vi "Measurement UI.vi"() -> ()   [LabVIEW 2021, in "crosstalk_Audio ADC.lvlib"]
uses:
  crosstalk_Audio ADC.lvlib
panel:
  out "MeasTable":string[][](table)
  in  "MeasGraphs":T1(tab)=enum."Time Domain"
  out "FreqDomainGraph":cluster{"f0":dbl, "df":dbl, "Spectrum":dbl[]}[](graph) caption="AC"
  out "TimeDomainGraph":waveform(dbl)[](graph) caption="AC"
  out "Time domain plot size":i32
  out "Spectrum plot size":i32
  out "dt":dbl
  out "t0":dbl
  out "df":dbl
  out "f0":dbl
  out "Time domain":dbl[](array[numeric])
  out "Spectrum":dbl[](array[numeric])
  out "Frequency 2":dbl
  out "Crosstalk":dbl
  out "Victim channel name":string
  out "Crosstalk waveform":dbl[](array[numeric])
  out "Frequency waveform":dbl[](array[numeric])
  in  "Victim channel resource name":string
  in  "Digital capture resource name":string
  in  "Configuration tab":enum32{"Protocol", "Measurement"}(tab)=enum."Measurement"
  in  "Frame sync edge for Channel 0":enum16{"Rising", "Falling"}(ring)=enum."Falling"
  in  "Channel count per frame":u8=2
  in  "Channel length":u16=32
  in  "Bit depth":u8=24
  in  "Channel 0 offset":u16=1
  in  "Endianness":enum16{"MSB First", "LSB First"}(ring)
  in  "Data Justification":enum16{"Left Justified", "Right Justified"}(ring) caption="Data justification"
  in  "Frame length":u16=64
  in  "Frame sync pulse width":u16=32
  in  "Bit clock edge sync":enum8{"Rising", "Falling"}(ring)=enum."Falling"
  in  "I2S":bool
  in  "LJ":bool
  in  "RJ":bool
  in  "TDM":bool
  in  "Analog source resource name":string(combo) caption="Resource Name"
  in  "Protocol capture resource name":string(combo) caption="Resource Name"
  in  "Channel Name":string
  in  "Full scale range":dbl=2.825 caption="FULL SCALE RANGE" format="%.3pV"
  in  "Weighting Filter":string(combo)="Linear"
  in  "Data line":u16 caption="Data Line"
  in  "Sample rate":dbl=44100.0 caption="Sample Rate" format="%#.6pHz"
  in  "Measurement settings":string="Measurement Settings"
  in  "Victim amplitude":dbl=1.0 caption="Amplitude" format="%#_6pdB"
  in  "Frequency":dbl=1000.0 format="%#_6pHz"
  in  "Victim channel":dbl=1.0 caption="Vicitim Channel" format="%#_6p"
  in  "Interferer channel":dbl caption="Interferer Channel" format="%#_6p"
  in  "Analog source":string="Analog source"
  in  "Digital capture":string="Digital capture"
  # "Protocols"
  # "PCM data configuration"
  # "Frame sync clock control"
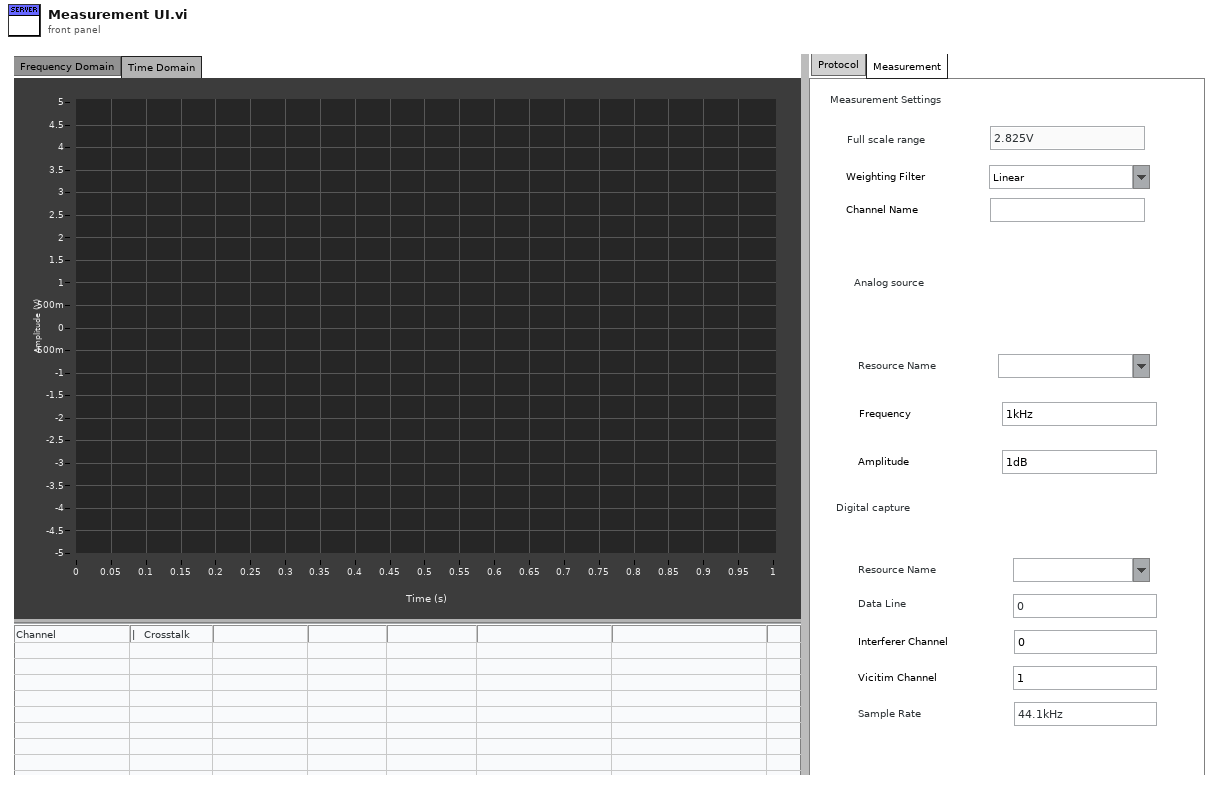
[diagram p1: front panel]
types:
  T1 = enum32{"Frequency Domain", "Time Domain", "Hidden Controls"}
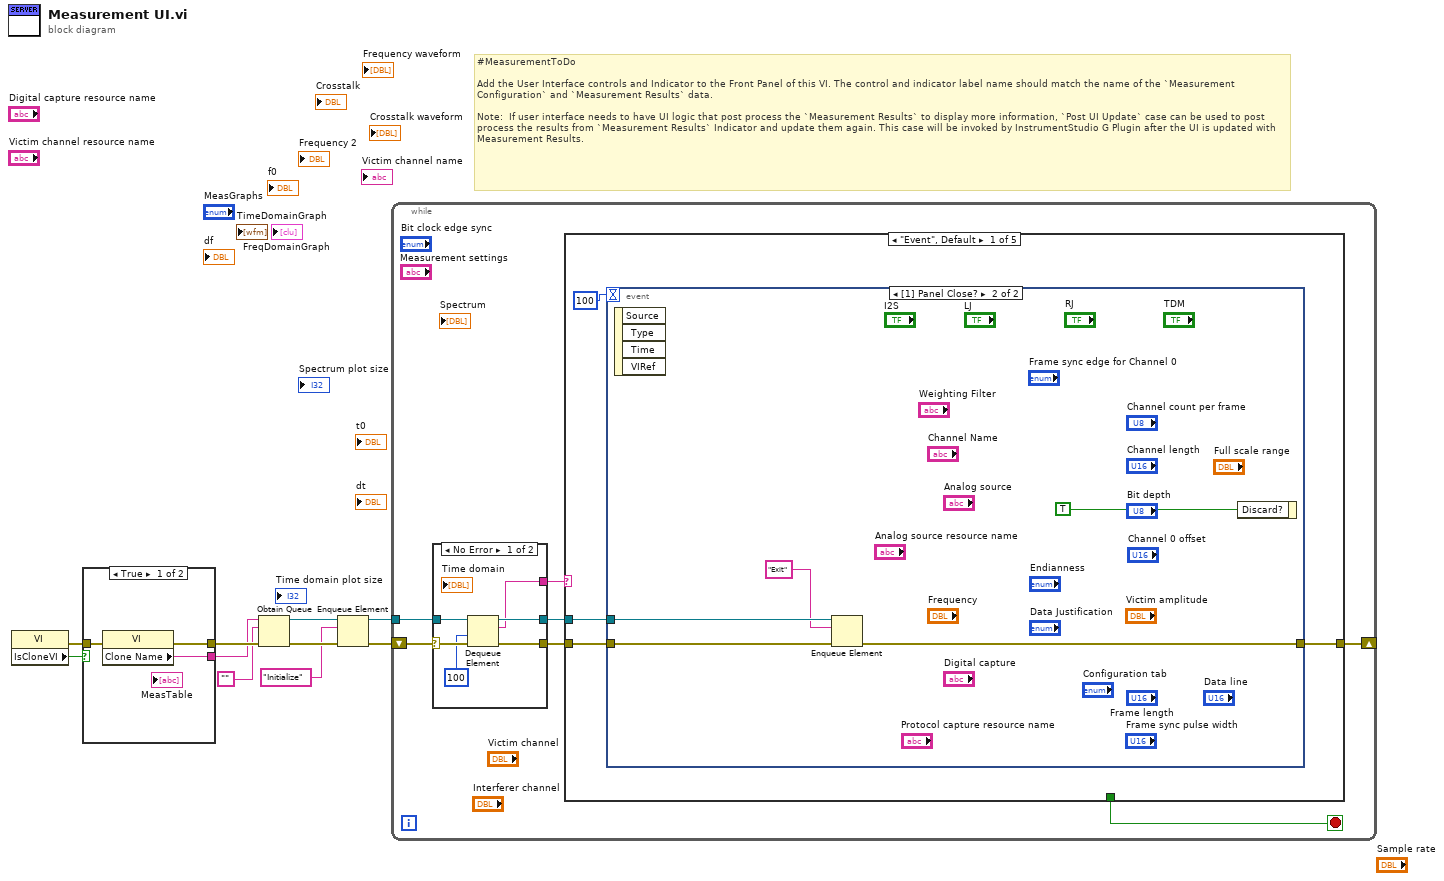
[diagram p0: block diagram]
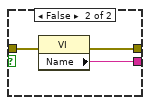
[diagram p2: hidden frame]
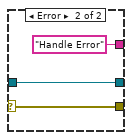
[diagram p3: hidden frame]
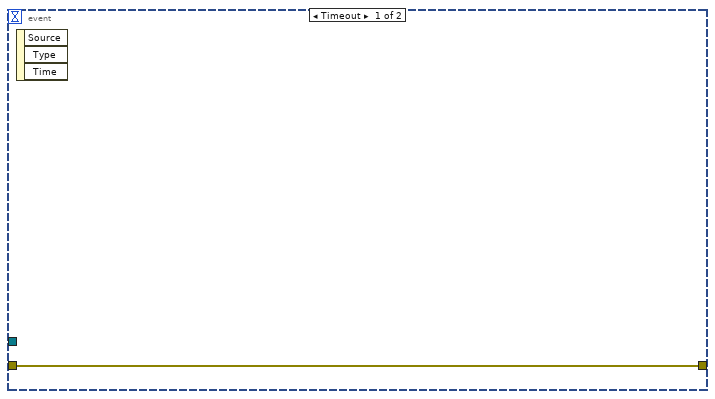
[diagram p4: hidden frame]
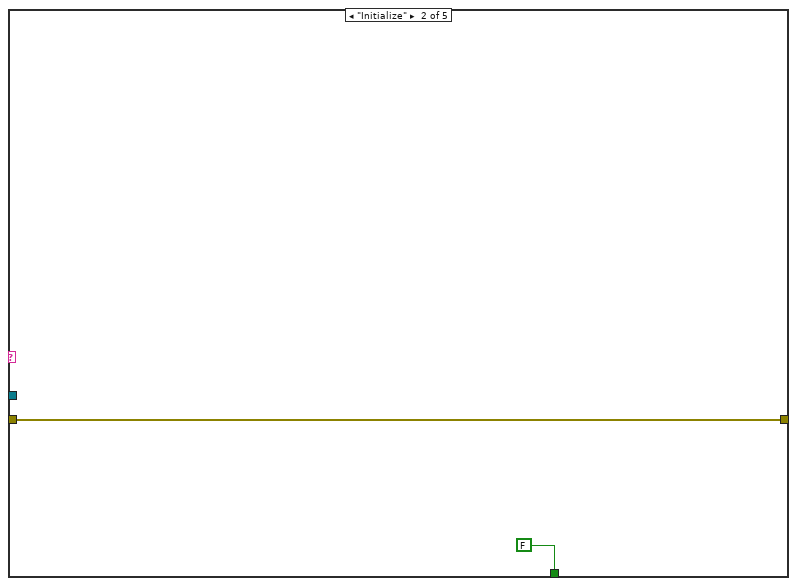
[diagram p5: hidden frame]
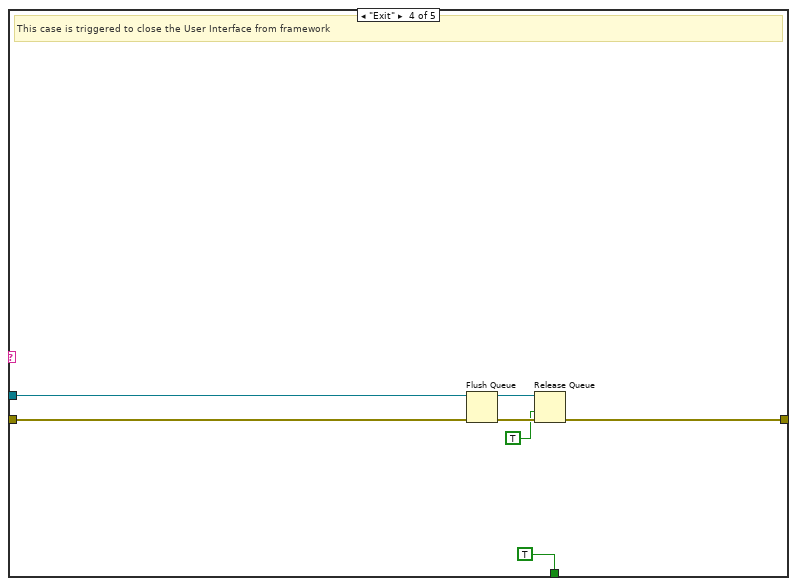
[diagram p7: hidden frame]
diagram:
  # "#MeasurementToDo  \n\nAdd the User Interface controls and Indicator to the Front Panel of this VI. The control and indicator label name should match the name of the `Measurement Configuration` and `Measurement Results` data.\n\nNote:  If user interface needs to have UI logic that post process the `Measurement Results` to display more information, `Post UI Update` case can be used to post process the results from `Measurement Results` Indicator and update them again. This case will be invoked by InstrumentStudio G Plugin after the UI is updated with Measurement Results."
  n1 = property class="VI"() -> (error out=w1:errorcluster, "IsCloneVI"=w2:bool)  [unwired: 2 in, 1 out]
  n2 = case shown="True" w2 {
    tunnel: [w13 w16] -> w10
    tunnel: [w12 w15] -> w9
    tunnel: w1 -> [w11 w14]
    frame True {
      n3 = property class="VI"(error in=w11) -> (error out=w13:errorcluster, "Clone Name"=w12:string)  [unwired: 1 in, 1 out]
    }
    frame False {
      n4 = property class="VI"(error in=w14) -> (error out=w16:errorcluster, "Name"=w15:string)  [unwired: 1 in, 1 out]
    }
  }
  n5 = Obtain Queue(name (unnamed)=w9, element data type="", error in (no error)=w10) -> (queue out=w6:refnum<queue>, error out=w8:errorcluster)  [unwired: 2 in, 1 out]
  n6 = Enqueue Element(queue=w6, element="Initialize", error in (no error)=w8) -> (queue out=w5:refnum<queue>, error out=w7:errorcluster)  [unwired: 1 in, 1 out]
  n7 = while {
    shift-right: [w18] -> _
    shift-left: w7 -> [w23]
    tunnel: w5 -> [w21]
    stop <- w17 stop-if-true
    n8 = case shown="No Error" w23 {
      selector: w23 -> [w29 w32]
      tunnel: [w28 w32] -> w22
      tunnel: w21 -> [w27 w31]
      tunnel: [w26 w31] -> w20
      tunnel: [w25 "Handle Error"] -> w19
      frame No Error {
        n9 = Dequeue Element(queue=w27, timeout in ms (-1)=100, error in (no error)=w29) -> (queue out=w26:refnum<queue>, element=w25:string, error out=w28:errorcluster)  [unwired: 1 out]
      }
      frame Error {
      }
    }
    n10 = case shown="\"Event\", Default" w19 {
      tunnel: w22 -> [w35 w44 w45 w52 w53]
      tunnel: w20 -> [w33 _ _ w50 _]
      tunnel: [w36 w44 w45 w47 w53] -> w18
      tunnel: [_ FALSE _ TRUE _] -> w17
      frame "Event", Default {
        n11 = event shown="[1] Panel Close?" {
          selector: _ -> [_ _]
          dyn-events: _ -> [_ _]
          timeout: 100 -> [_ _]
          tunnel: [w37 w40] -> w36
          tunnel: w35 -> [w37 w41]
          tunnel: w33 -> [_ w39]
          event Timeout {
            n12 = event-data() -> ()  [unwired: 1 in, 3 out]
          }
          event Panel Close? {
            n13 = event-data() -> ()  [unwired: 1 in, 4 out]
            n14 = Enqueue Element(queue=w39, element="Exit", error in (no error)=w41) -> (error out=w40:errorcluster)  [unwired: 1 in, 2 out]
            n15 = event-data("Discard?"=TRUE) -> ()  [unwired: 1 in, 1 out]
          }
        }
      }
      frame "Initialize" {
      }
      frame "Post UI Update" {
        # "This case will be triggered, after framework updates the User interface with result values."
      }
      frame "Exit" {
        # "This case is triggered to close the User Interface from framework"
        n16 = Flush Queue(queue=w50, error in (no error)=w52) -> (queue out=w49:refnum<queue>, error out=w48:errorcluster)  [unwired: 1 out]
        n17 = Release Queue(queue=w49, force destroy? (F)=TRUE, error in (no error)=w48) -> (error out=w47:errorcluster)  [unwired: 2 out]
      }
      frame "Handle Error" {
      }
    }
  }
